vi "Read_FFID_Auto_Calib_Setup.vi"(5 "Specific Argument":string) -> (0 "Trace concentration %":dbl[](array[numeric]), 1 "Carrier 2 Q":dbl[](array[numeric]), 2 "Carrier 1 Q":dbl[](array[numeric]), 3 "Mix_own_Calib_Gases":bool, 4 "Error String":string)   [LabVIEW 2022 SP3]
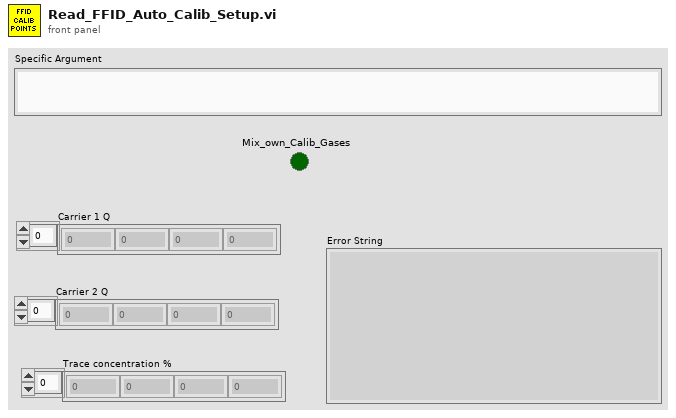
[diagram p1: front panel]
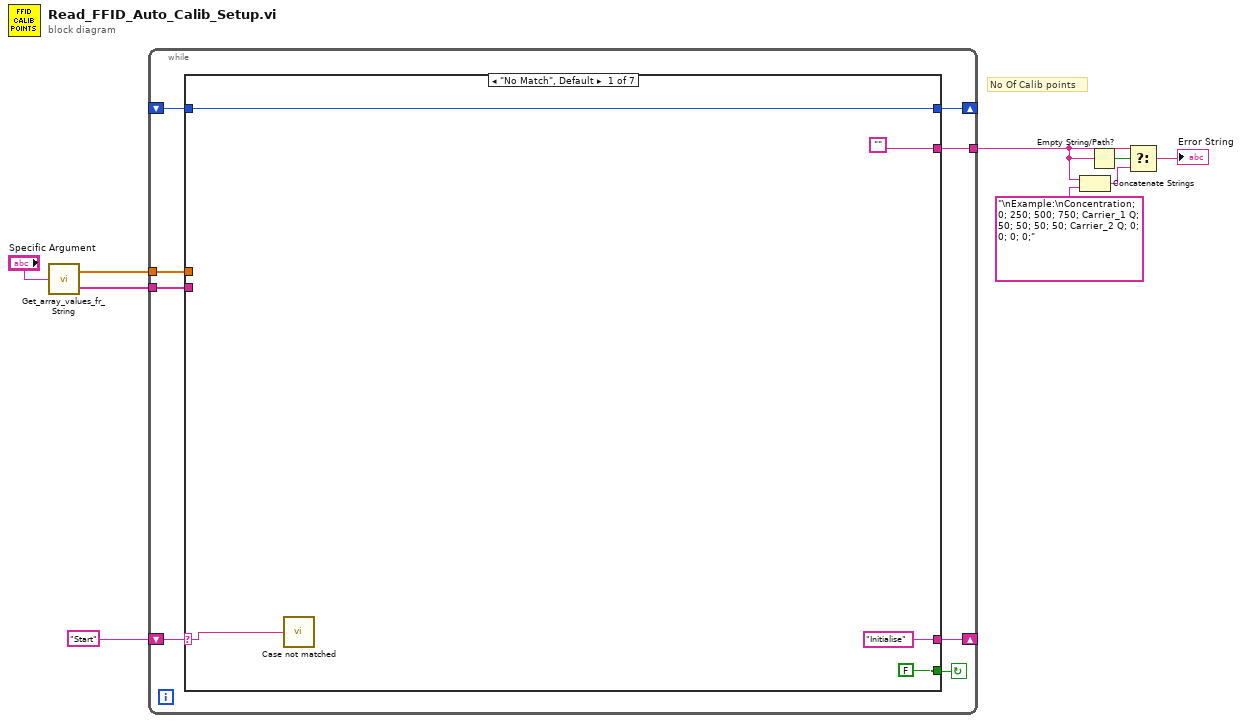
[diagram p0: block diagram]
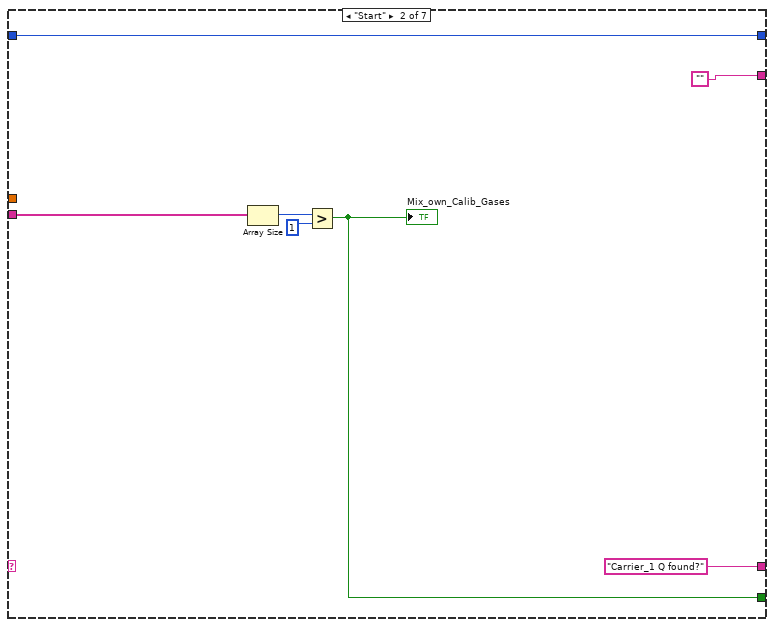
[diagram p2: hidden frame]
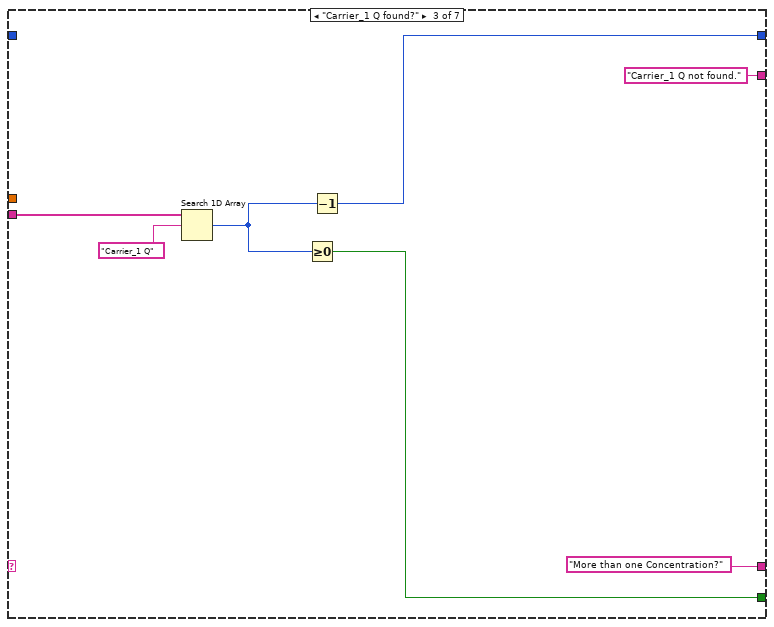
[diagram p3: hidden frame]
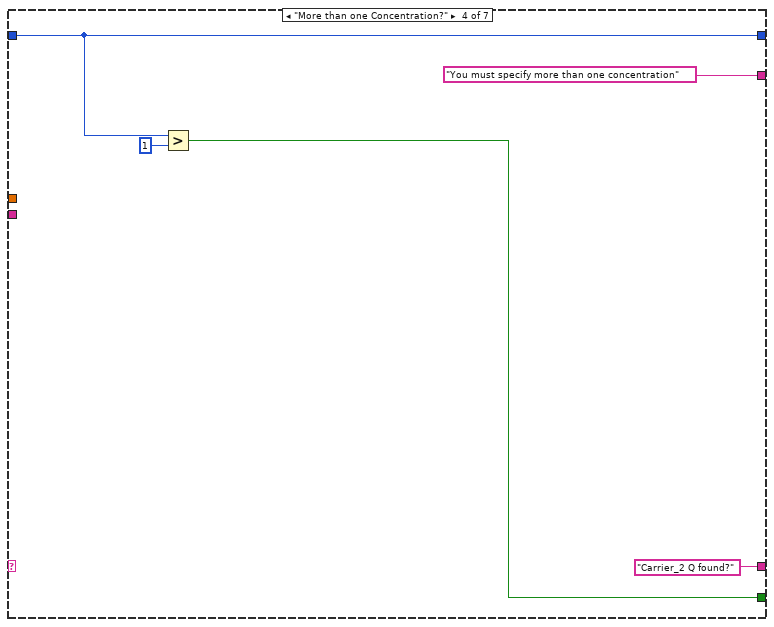
[diagram p4: hidden frame]
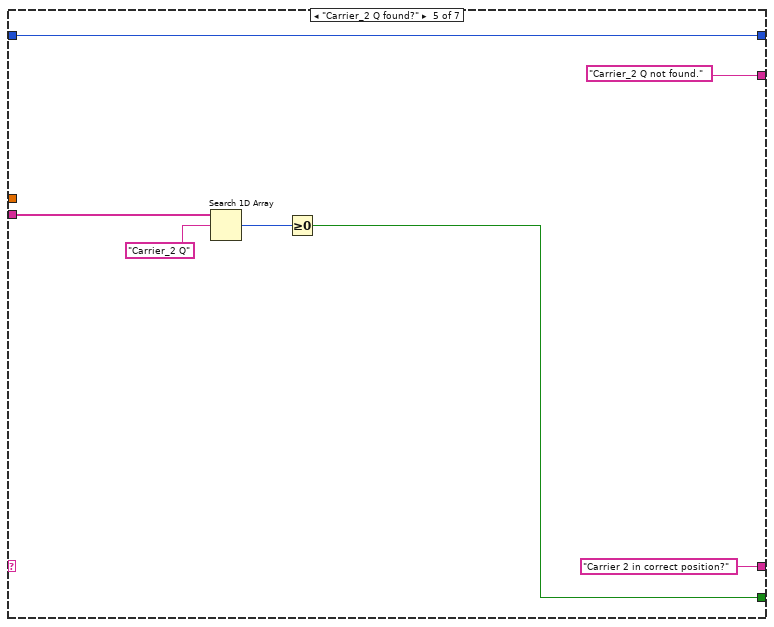
[diagram p5: hidden frame]
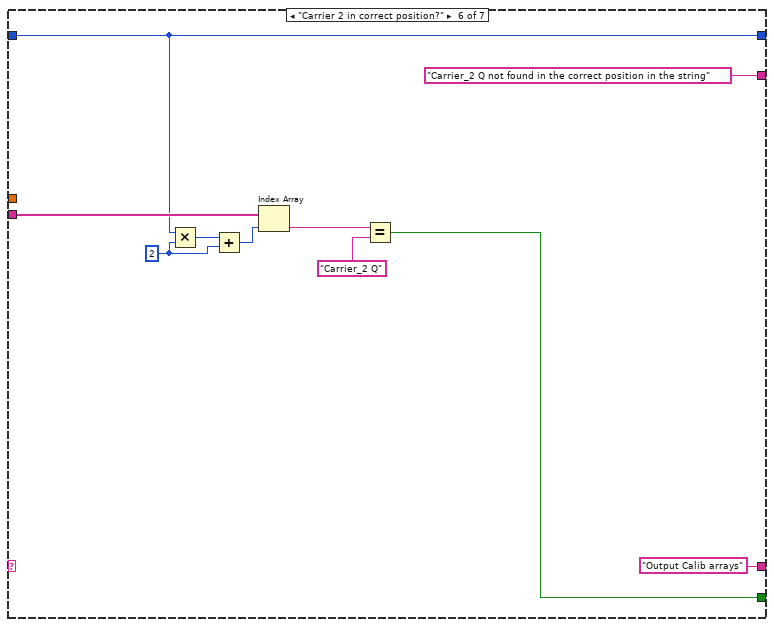
[diagram p6: hidden frame]
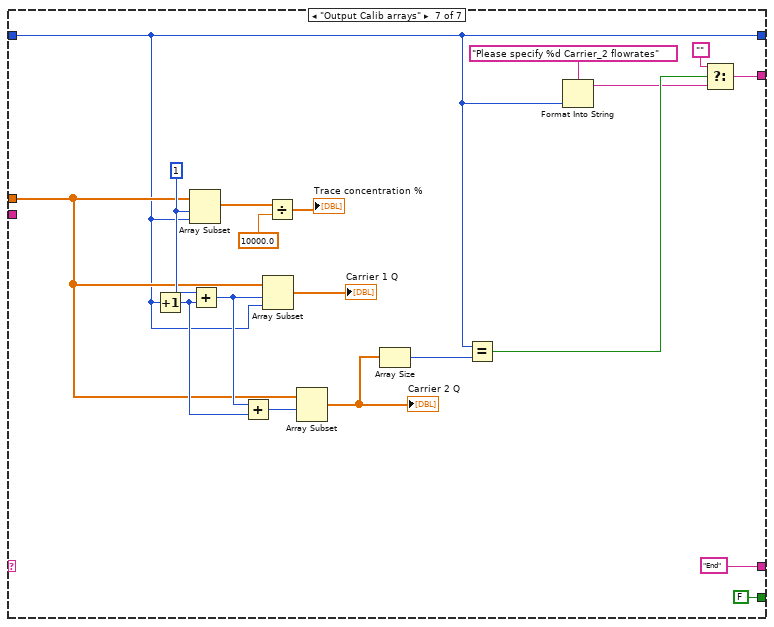
[diagram p7: hidden frame]
diagram:
  # "No Of Calib points"
  n1 = call "Get_array_values_fr_String.vi"("String Value"="Specific Argument") -> ("Numeric Array"=w6:dbl[], "String array"=w7:string[])
  n2 = while {
    shift-left: "Start" -> [w15]
    shift-right: [w16] -> _
    tunnel: w7 -> [w14]
    tunnel: [w13] -> w3
    shift-right: [w12] -> _
    shift-left: _ -> [w11]
    tunnel: w6 -> [w10]
    stop <- w17 continue-if-true
    n3 = case shown="\"No Match\", Default" w15 {
      selector: w15 -> [w18 _ _ _ _ _ _]
      tunnel: [FALSE w25 w33 w37 w42 w54 FALSE] -> w17
      tunnel: ["Initialise" "Carrier_1 Q found?" "More than one Concentration?" "Carrier_2 Q found?" "Carrier 2 in correct position?" "Output Calib arrays" "End"] -> w16
      tunnel: w14 -> [_ w26 w34 _ w46 w57 _]
      tunnel: ["" "" "Carrier_1 Q not found." "You must specify more than one concentration" "Carrier_2 Q not found." "Carrier_2 Q not found in the correct position in the string" w63] -> w13
      tunnel: [w20 w23 w30 w38 w45 w56 w61] -> w12
      tunnel: w11 -> [w20 w23 _ w38 w45 w56 w61]
      tunnel: w10 -> [_ _ _ _ _ _ w72]
      frame "No Match", Default {
        n4 = call "Case not matched.vi"("Case Name not Matched"=w18) -> ()
      }
      frame "Start" {
        n5 = Array Size(array=w26) -> (size(s)=w28:i32)
        n6 = Greater?(x=w28, y=1) -> (0:w25:bool)
        "Mix_own_Calib_Gases" <- w25
      }
      frame "Carrier_1 Q found?" {
        n7 = Search 1D Array(1D array=w34, element="Carrier_1 Q") -> (index of element=w31:i32)  [unwired: 1 in]
        n8 = Greater Or Equal To 0?(x=w31) -> (x >= 0?=w33:bool)
        n9 = Decrement(x=w31) -> (x-1=w30:i32)
      }
      frame "More than one Concentration?" {
        n10 = Greater?(x=w38, y=1) -> (0:w37:bool)
      }
      frame "Carrier_2 Q found?" {
        n11 = Search 1D Array(1D array=w46, element="Carrier_2 Q") -> (index of element=w47:i32)  [unwired: 1 in]
        n12 = Greater Or Equal To 0?(x=w47) -> (x >= 0?=w42:bool)
      }
      frame "Carrier 2 in correct position?" {
        w50 = 2 ("y")
        n13 = Multiply(x=w56, y=w50) -> (x*y=w51:i32)
        n14 = Add(x=w51, y=w50) -> (x+y=w49:i32)
        n15 = Index Array(array=w57, index=w49) -> (element=w55:string)
        n16 = Equal?(x=w55, y="Carrier_2 Q" ("element")) -> (x = y?=w54:bool)
      }
      frame "Output Calib arrays" {
        w76 = 1 ("index")
        n17 = Increment(x=w61) -> (x+1=w74:i32)
        n18 = Array Subset(array=w72, index=w76, length=w61) -> (w71:dbl[])
        n19 = Add(x=w76, y=w74) -> (x+y=w75:i32)
        n20 = Add(x=w75, y=w74) -> (x+y=w73:i32)
        n21 = Array Subset(array=w72, index=w75, length=w61) -> (→"Carrier 1 Q":dbl[])
        n22 = Divide(x=w71, y=10000.0) -> (x/y=→"Trace concentration %":dbl[])
        n23 = Array Subset(array=w72, index=w73) -> (w68:dbl[])  [unwired: 1 in]
        "Carrier 2 Q" <- w68
        n24 = Array Size(array=w68) -> (size(s)=w65:i32)
        n25 = Equal?(x=w61, y=w65) -> (x = y?=w62:bool)
        n26 = Format Into String(format string="Please specify %d Carrier_2 flowrates", w61) -> (resulting string=w59:string)  [unwired: 2 in, 1 out]
        n27 = Select(t="", s=w62, f=w59) -> (s? t:f=w63:string)
      }
    }
  }
  n28 = Concatenate Strings(w3, "\nExample:\nConcentration; 0; 250; 500; 750; Carrier_1 Q; 50; 50; 50; 50; Carrier_2 Q; 0; 0; 0; 0;") -> (w2:string)
  n29 = Empty String/Path?(string/path=w3) -> (empty?=w5:bool)
  n30 = Select(t=w3, s=w5, f=w2) -> (s? t:f=→"Error String":string)
